vi "gxml_GetArrayElementInfo.vi"(6 "Item Data":T1, 7 "XML Array Empty?":bool, 8 "error in":errorcluster, 9 "Flat String In":string, 11 "Array TypeDesc":variant) -> (0 "error out":errorcluster, 1 "Flat String Out":string, 2 "XML Array Empty?":bool, 3 "Element TypeDesc":variant, 5 "Element Count":i32)   [LabVIEW 2011, in "Third Party VIs.lvlib" / "GXML.lvlib"]
doc: "Accepting an Array Type Descriptor, this VI adds the header information to the Running Flattened String, and extracts the Type Descriptor of the array elements.\n\nIn parallel, the VI also pulls header information from the default data flattened string. If the XML file does not contain the array name being searched, then the header information from the default data is used.\n\nSubsequently, if array name is found in the XML file and its attribute dimensions do not match the dimenstions of of the type definition, an error is generated."
uses:
  GXML.lvlib
  <vilib>/Utility/VariantDataType/VariantType.lvlib
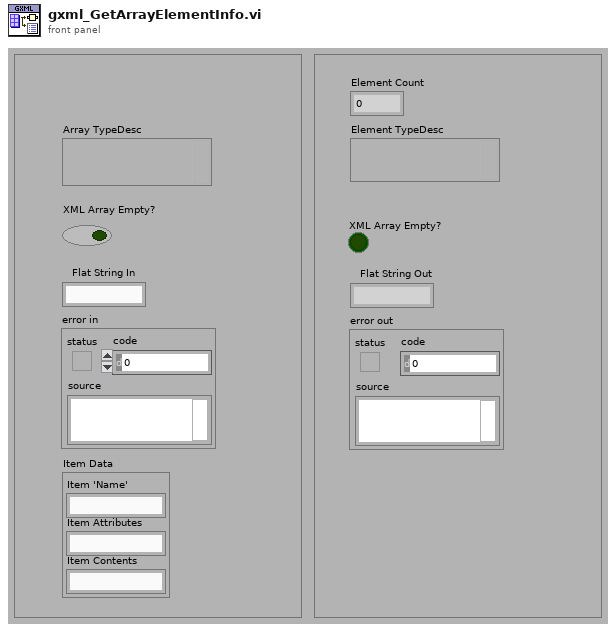
[diagram p1: front panel]
types:
  T1 = cluster{"Item 'Name'":string, "Item Attributes":string, "Item Contents":string}
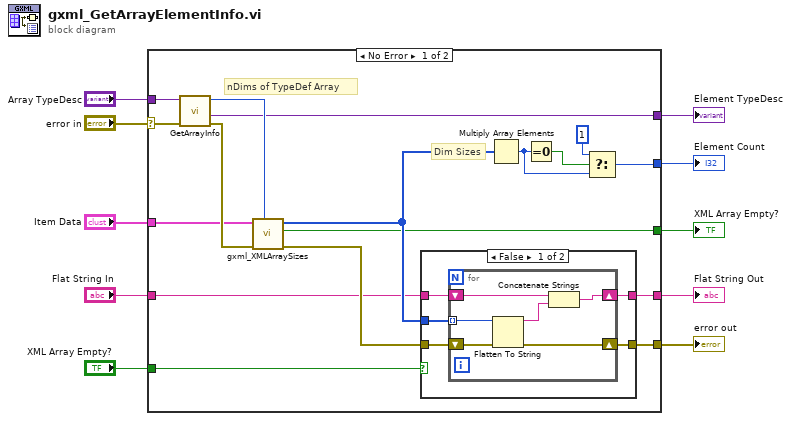
[diagram p0: block diagram]
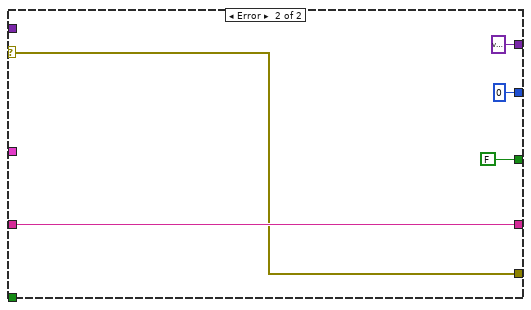
[diagram p3: hidden frame]
diagram:
  n1 = case shown="No Error" "error in" {
    selector: "error in" -> [w12 w41]
    tunnel: "Array TypeDesc" -> [w23 _]
    tunnel: [w21 variant ("ArrayElement")] -> w9
    tunnel: [w20 0 ("t")] -> w8
    tunnel: [w19 w41] -> w7
    tunnel: "Item Data" -> [w16 _]
    tunnel: [w15 FALSE ("XML Array Empty?")] -> w5
    tunnel: "Flat String In" -> [w14 w42]
    tunnel: [w13 w42] -> w3
    tunnel: "XML Array Empty?" -> [w11 _]
    frame No Error {
      # "Dim Sizes"
      # "nDims of TypeDef Array"
      n2 = call <vilib>:"GetArrayInfo.vi"("error in (no error)"=w12, "Variant"=w23) -> ("error out"=w17:errorcluster, "ArrayElement"=w21:variant, "NDims"=w24:i32)  [unwired: 6 in, 1 out]
      n3 = call "gxml_XMLArraySizes.vi"("NDims"=w24, "error in"=w17, "Item Data"=w16) -> ("error out"=w18:errorcluster, "XML Array Empty?"=w15:bool, "Dim Sizes"=w22:i32[])  [unwired: 6 in]
      n4 = case shown="False" w11 {
        tunnel: w22 -> [w32 _]
        tunnel: [w31 w39] -> w19
        tunnel: w18 -> [w30 w39]
        tunnel: w14 -> [w29 w40]
        tunnel: [w28 w40] -> w13
        frame False {
          n5 = for {
            shift-right: [w37] -> w31
            shift-left: w30 -> [w38]
            shift-right: [w33] -> w28
            shift-left: w29 -> [w34]
            tunnel: w32 -> [w36] mode=indexing
            n6 = Flatten To String(anything=w36, error in (no error)=w38) -> (data string=w35:string, error out=w37:errorcluster)  [unwired: 2 in, 1 out]
            n7 = Concatenate Strings(w34, w35) -> (w33:string)
          }
        }
        frame True {
        }
      }
      n8 = Multiply Array Elements(1:w22) -> (0:w27:i32)
      n9 = Equal To 0?(x=w27) -> (x = 0?=w25:bool)
      n10 = Select(t=1, s=w25, f=w27) -> (s? t:f=w20:i32)
    }
    frame Error {
    }
  }
  "error out" <- w7
  "Element TypeDesc" <- w9
  "Element Count" <- w8
  "XML Array Empty?" <- w5
  "Flat String Out" <- w3
